vi "NI_FPGA_PPG.ProcConstructor.vi"(0 "i ref in":refnum<vi>, 3 "ms timeout (10000)":i32=10000, 5 "error in (no error)":errorcluster) -> (14 "i ref out":refnum<vi>, 17 "timed out":bool, 19 "error out":errorcluster)   [LabVIEW 2014, in "NI_FPGA_PPG.lvlib"]
doc: "This method provides some code that needs to be called while executing the constructor."
uses:
  NI_FPGA_PPG.lvlib
  CSCore/CSApplicationBaseClasses/DeviceBase/DeviceBase.lvlib
  CSinstr.lib/NI-FPGA-PPG/host/instrumentDriver/NI-FPGA_PPG_Driver.lvlib
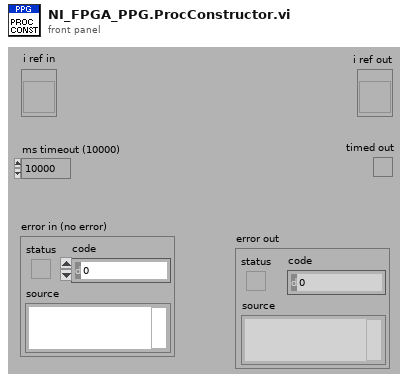
[diagram p1: front panel]
types:
  T1 = typedef "NI_FPGA_PPG.lvlib/NI_FPGA_PPG.i attribute.ctl" = cluster{"dim_service_id":cluster{"dim_actual_device_status":i32, "dim_event_data":i32, "dim_cmd_data":i32, "dim_cmd_data _description":i32, "dim_channel_description":i32}, "VISA":refnum<visa-resource-name>, "actual_device_status":i32, "event_data_id":i32, "pdc_enabled":bool, "pdc_timestamp":u32, "cmd_data_string":string, "cmd_data_size":i32, "cmd_data_description_string":string, "cmd_data_description_size":i32, "channel_description_string":string, "channel_description_size":i32}
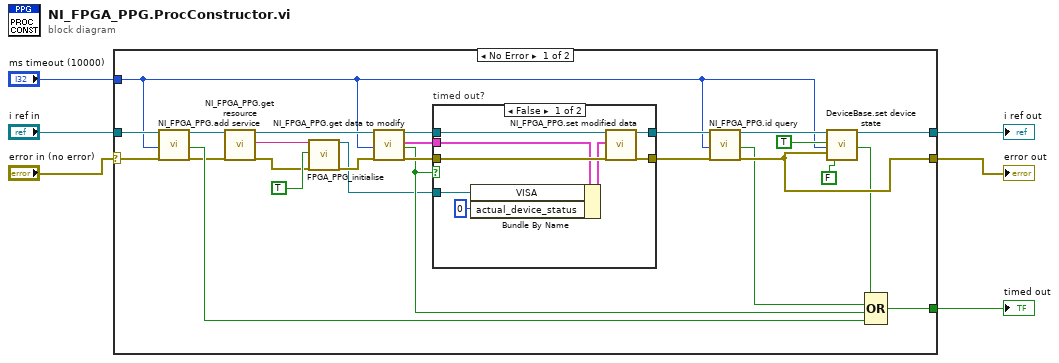
[diagram p0: block diagram]
diagram:
  n1 = case shown="No Error" "error in (no error)" {
    selector: "error in (no error)" -> [w21 w43]
    tunnel: "i ref in" -> [w20 w44]
    tunnel: [w26 w44] -> w4
    tunnel: [w12 w43] -> w3
    tunnel: "ms timeout (10000)" -> [w9 _]
    tunnel: [w22 _] -> w1
    frame No Error {
      n2 = call "NI_FPGA_PPG.add service.vi"("i ref in"=w20, "ms timeout (10000)"=w9, "error in (no error)"=w21) -> ("i ref out"=w17:refnum<vi>, "timed out"=w19:bool, "error out"=w18:errorcluster)  [unwired: 14 in]
      n3 = call "NI_FPGA_PPG.get resource.vi"("i ref in"=w17, "error in (no error)"=w18) -> ("i ref out"=w31:refnum<vi>, "resource"=w14:string, "error out"=w28:errorcluster)  [unwired: 15 in]
      n4 = call "FPGA_PPG_initialise.vi"("resource_in"=w14, "reset"=TRUE, "error in (no error)"=w28) -> ("resource_out"=w15:refnum<visa-resource-name>, "error out"=w16:errorcluster)  [unwired: 14 in, 1 out]
      n5 = call "NI_FPGA_PPG.get data to modify.vi"("i ref in"=w31, "ms timeout (10000)"=w9, "error in (no error)"=w16) -> ("i ref out"=w29:refnum<vi>, "i attribute"=w27:T1, "timed out"=w23:bool, "error out"=w30:errorcluster)  [unwired: 13 in]
      n6 = case "timed out?" shown="False" w23 {
        tunnel: w30 -> [w40 w41]
        tunnel: w29 -> [w39 w42]
        tunnel: [w38 w42] -> w11
        tunnel: [w37 w41] -> w13
        tunnel: w27 -> [w36 _]
        tunnel: w15 -> [w34 _]
        frame False {
          n7 = Bundle By Name(cluster=w36, "VISA"=w34, "actual_device_status"=0) -> (w35:T1)
          n8 = call "NI_FPGA_PPG.set modified data.vi"("i ref in"=w39, "i attribute"=w35, "error in (no error)"=w40) -> ("i ref out"=w38:refnum<vi>, "error out"=w37:errorcluster)  [unwired: 15 in]
        }
        frame True {
        }
      }
      n9 = call "NI_FPGA_PPG.id query.vi"("i ref in"=w11, "ms timeout (10000)"=w9, "error in (no error)"=w13) -> ("i ref out"=w10:refnum<vi>, "timed out"=w7:bool, "error out"=w12:errorcluster)  [unwired: 13 in, 1 out]
      n10 = call "DeviceBase.set device state.vi"("i ref in"=w10, "implicit"=TRUE, "ms timeout (10000)"=w9, "device error"=w12, "mayResetError (FALSE)"=FALSE) -> ("i ref out"=w26:refnum<vi>, "timed out"=w8:bool)  [unwired: 12 in, 1 out]
      n11 = Compound Arithmetic op=OR(w8, w7, w23, w19) -> (w22:bool)
    }
    frame Error {
    }
  }
  "error out" <- w3
  "i ref out" <- w4
  "timed out" <- w1
